vi "Set Selected Application Instance.vi"(10 "Application out":refnum<vi>, 11 "Configuration":T1) -> (3 "ConfigurationOut":T1={"Data Tree Ref"=refnum, "FP Ref"=refnum, "Column Data Type"=[], "Search Clones Up To"=100, "SortOptions"={"Col.pri"=0, "RevDir.pri"=FALSE, "Col.sec"=0, "RevDir.sec"=FALSE}, "Group/Flat (0:group)"=FALSE, "CollapsedNodes"=[], "Show/Hide Cols"=[], "Filtered Paths"=[], "View"=enum."Group By Library", "File Extension Filters"=[], "Filter Global VIs"=FALSE, "Shared"=refnum, "Active Filters"=refnum, "Refresh Rate (ms)"=2000, "App Instance Ring Ref"=refnum, "Processing Q"=refnum, "VI Ref"=refnum})   [LabVIEW 2013, in "LVTM.lvlib"]
uses:
  LVTM.lvlib
  Controls_LVTM/View.ctl
  Controls_LVTM/SharedDataDVR.ctl
  Controls_LVTM/LVTM_Config_Info.ctl
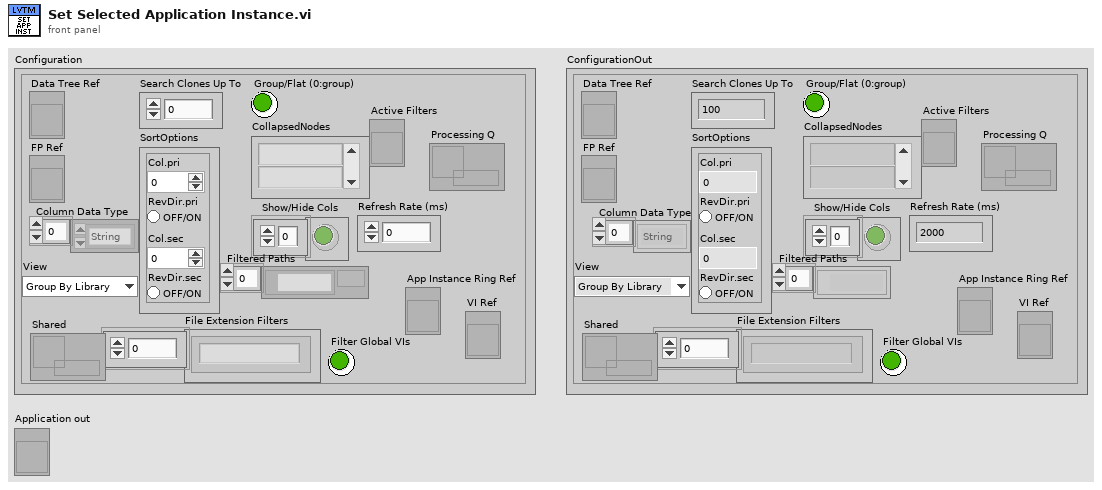
[diagram p1: front panel]
types:
  T1 = typedef "LVTM.lvlib/LVTM_Config_Info.ctl" = cluster{"Data Tree Ref":refnum<vi>, "FP Ref":refnum<vi>, "Column Data Type":enum16{"String", "Numeric"}[], "Search Clones Up To":i32, "SortOptions":cluster{"Col.pri":i32, "RevDir.pri":bool, "Col.sec":i32, "RevDir.sec":bool}, "Group/Flat (0:group)":bool, "CollapsedNodes":string[], "Show/Hide Cols":bool[], "Filtered Paths":path[], "View":T2, "File Extension Filters":string[], "Filter Global VIs":bool, "Shared":refnum<data-value>, "Active Filters":refnum<vi>, "Refresh Rate (ms)":i32, "App Instance Ring Ref":refnum<vi>, "Processing Q":refnum<queue>, "VI Ref":refnum<vi>}
  T2 = typedef "LVTM.lvlib/View.ctl" = enum16{"Group By Library", "Group By Folder", "Flat List"}
  T3 = typedef "LVTM.lvlib/SharedDataDVR.ctl" = cluster{"App":refnum<vi>, "VIs":string[]}
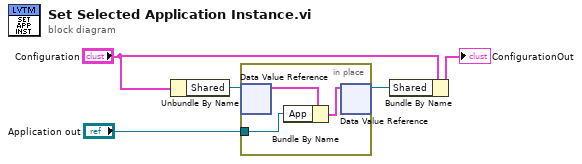
[diagram p0: block diagram]
diagram:
  n1 = Unbundle By Name("Configuration") -> ("Shared"=w5:refnum<data-value>)
  n2 = in-place {
    in-place-border: "Application out" -> [w6]
    n3 = in-place-dvr #1(w5) -> (w8:T3)  [unwired: 1 out]
    n4 = Bundle By Name(cluster=w8, "App"=w6) -> (w7:T3)
    n5 = in-place-dvr #1(w7) -> (w3:refnum<data-value>)  [unwired: 1 out]
  }
  n6 = Bundle By Name(cluster="Configuration", "Shared"=w3) -> (→"ConfigurationOut":T1)
